vi "Report Analog Command.vi"(6 "Value":dbl, 8 "error in (no error)":errorcluster, 9 "Name":string, 10 "VolatusAPI in":refnum<class "VolatusAPI.lvclass">, 11 "GUI Element in":refnum<class "GUI Element.lvclass">) -> (0 "error out":errorcluster, 3 "GUI Element out":refnum<class "GUI Element.lvclass">)   [LabVIEW 2020, in "VolatusGUI.lvlib" / "GUI Element.lvclass"]
uses:
  GUI Element.lvclass
  Volatus/VolatusAPI/VolatusAPI.lvclass
  GUI Element.lvclass/GUI Element.ctl
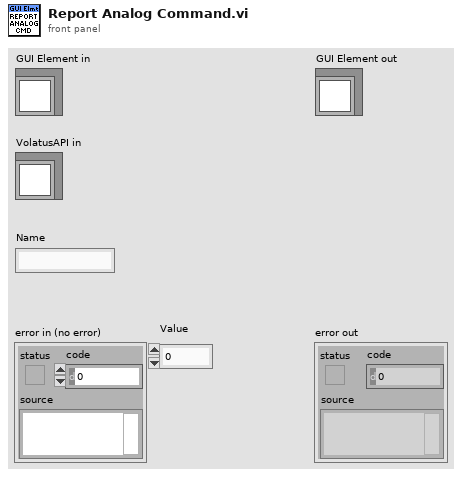
[diagram p1: front panel]
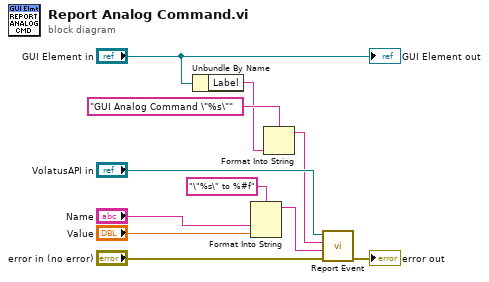
[diagram p0: block diagram]
diagram:
  n1 = Unbundle By Name("GUI Element in") -> ("Label"=w1:string)
  n2 = Format Into String(format string="\"%s\" to %#f", "Name", "Value") -> (resulting string=w4:string)  [unwired: 2 in, 1 out]
  n3 = Format Into String(format string="GUI Analog Command \"%s\"" ("string"), w1) -> (resulting string=w3:string)  [unwired: 2 in, 1 out]
  n4 = call "Report Event.vi"("error in (no error)"="error in (no error)", "Message"=w4, "Context"=w3, "VolatusAPI in"="VolatusAPI in") -> ("error out"=→"error out":errorcluster)  [unwired: 6 in, 1 out]
  "GUI Element out" <- "GUI Element in"
